vi "I_regulering.vi"(9 "k_i":dbl, 10 "SP":dbl, 11 "DATA":dbl) -> (1 "i_i":dbl, 2 "e(t)":dbl, 3 "u_i":dbl)   [LabVIEW 2022 SP3]
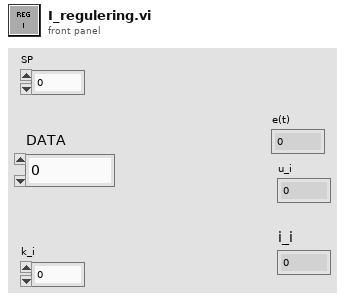
[diagram p1: front panel]
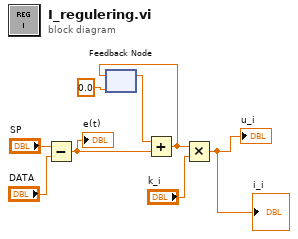
[diagram p0: block diagram]
diagram:
  n1 = Subtract(x="SP", y="DATA") -> (x-y=w4:dbl)
  "e(t)" <- w4
  n2 = feedback #1(0.0) -> (w5:dbl)
  n3 = Add(x=w5, y=w4) -> (x+y=w1:dbl)
  n4 = feedback-in #1(w1) -> ()
  n5 = Multiply(x=w1, y="k_i") -> (x*y=→"u_i" →"i_i":dbl)
